vi "LL_POST Object (Core).vi"(7 "Data":string, 8 "error in (no error)":errorcluster, 9 "Bucket":string, 10 "Path":string="/", 11 "Headers":T2[](array[typedef])) -> (0 "error out":errorcluster, 1 "Call Result":T1, 2 "Response body":string, 3 "Response header":string)   [LabVIEW 2011, in "LV Interface for Amazon S3.lvlib"]
doc: "This core implementation of the POST operation may be used to implement special requests or API calls not present in this toolkit. POST Object operation adds an object to a specified bucket using HTML forms. POST is an alternate form of PUT that enables browser-based uploads as a way of putting objects in buckets. Parameters that are passed to PUT via HTTP Headers are instead passed as form fields to POST in the multipart/form-data encoded message body."
uses:
  LV Interface for Amazon S3.lvlib
  Typedefs/AMZ_S3_HTTP Header-Value pair.ctl
  Typedefs/AMZ_S3_Call Results.ctl
  <vilib>/httpClient/POSTBuffer.vi
  <vilib>/httpClient/LabVIEWHTTPClient.lvlib
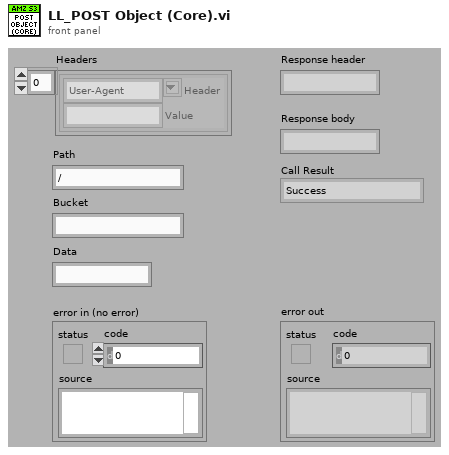
[diagram p1: front panel]
types:
  T1 = typedef "LV Interface for Amazon S3.lvlib/AMZ_S3_Call Results.ctl" = enum16{"Success", "UndefinedError", "AccessDenied", "AccountProblem", "AmbiguousGrantByEmailAddress", "BadDigest", "BucketAlreadyExists", "BucketAlreadyOwnedByYou", "BucketNotEmpty", "CredentialsNotSupported", "CrossLocationLoggingProhibited", "EntityTooSmall", "EntityTooLarge", "ExpiredToken", "IllegalVersioningConfigurationException", "IncompleteBody", "IncorrectNumberOfFilesInPostRequest", "InlineDataTooLarge", "InternalError", "InvalidAccessKeyId", "InvalidAddressingHeader", "InvalidArgument", "InvalidBucketName", "InvalidDigest", "InvalidLocationConstraint", "InvalidPart", "InvalidPartOrder", "InvalidPayer", "InvalidPolicyDocument", "InvalidRange", "InvalidSecurity", "InvalidSOAPRequest", "InvalidStorageClass", "InvalidTargetBucketForLogging", "InvalidToken", "InvalidURI", "KeyTooLong", "MalformedACLError", "MalformedPOSTRequest", "MalformedXML", "MaxMessageLengthExceeded", "MaxPostPreDataLengthExceededError", "MetadataTooLarge", "MethodNotAllowed", "MissingAttachment", "MissingContentLength", "MissingRequestBodyError", "MissingSecurityElement", "MissingSecurityHeader", "NoLoggingStatusForKey", "NoSuchBucket", "NoSuchKey", "NoSuchUpload", "NoSuchVersion", "NotImplemented", "NotSignedUp", "OperationAborted", "PermanentRedirect", "PreconditionFailed", "Redirect", "RequestIsNotMultiPartContent", "RequestTimeout", "RequestTimeTooSkewed", "RequestTorrentOfBucketError", "SignatureDoesNotMatch", "SlowDown", "TemporaryRedirect", "TokenRefreshRequired", "TooManyBuckets", "UnexpectedContent", "UnresolvableGrantByEmailAddress", "UserKeyMustBeSpecified", "LabVIEWError"}
  T2 = typedef "LV Interface for Amazon S3.lvlib/AMZ_S3_HTTP Header-Value pair.ctl" = cluster{"Header":string, "Value":string}
  T3 = typedef "LabVIEWHTTPClient.lvlib/ClientHandle.ctl" = refnum<k1>
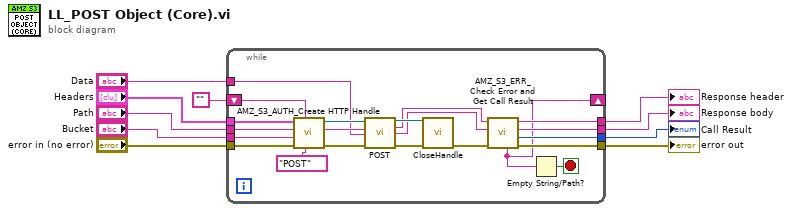
[diagram p0: block diagram]
diagram:
  n1 = while {
    tunnel: "Data" -> [w27]
    tunnel: "Headers" -> [w21]
    tunnel: "Path" -> [w20]
    tunnel: "Bucket" -> [w19]
    tunnel: "error in (no error)" -> [w18]
    tunnel: [w17] -> w5
    tunnel: [w16] -> w4
    tunnel: [w14] -> w3
    tunnel: [w15] -> w2
    shift-right: [w11] -> _
    shift-left: "" -> [w12]
    stop <- w13 stop-if-true
    n2 = call "AMZ_S3_AUTH_Create HTTP Handle.vi"("HTTP-Verb"="POST", "Redirect endpoint"=w12, "error in (no error)"=w18, "Bucket"=w19, "Path and query string"=w20, "Headers"=w21) -> ("error out"=w30:errorcluster, "URL"=w28:string, "client handle out"=w29:T3)  [unwired: 3 in]
    n3 = call-poly <vilib>:"POST.vi"("client handle"=w29, "url"=w28, "data"=w27, "error in (no error)"=w30) -> ("client handle out"=w25:T3, "headers"=w23:string, "body"=w22:string, "error out"=w26:errorcluster)  [unwired: 8 in]
    n4 = call <vilib>:"CloseHandle.vi"("client handle"=w25, "error in (no error)"=w26) -> ("error out"=w24:errorcluster)  [unwired: 13 in]
    n5 = call "AMZ_S3_ERR_Check Error and Get Call Result.vi"("error in (no error)"=w24, "Response body"=w22, "Response header"=w23) -> ("error out"=w15:errorcluster, "Call Result"=w14:T1, "Response body dup"=w16:string, "Response header dup"=w17:string, "Redirect endpoint"=w11:string)  [unwired: 4 in]
    n6 = Empty String/Path?(string/path=w11) -> (empty?=w13:bool)
  }
  "Response header" <- w5
  "Response body" <- w4
  "Call Result" <- w3
  "error out" <- w2
